vi "VI.OpenRef.caller.vi"(6 "options":i32, 8 "error in":errorcluster caption="error in (no error)", 9 "VI.ref":refnum<vi> caption="VI.ref ('caller' if not wired)") -> (0 "error out":errorcluster, 1 "VI.ref out":refnum<vi>, 4 "opened new?":bool)   [LabVIEW 2020]
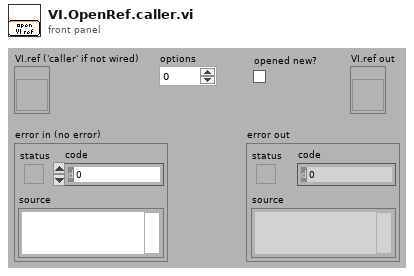
[diagram p1: front panel]
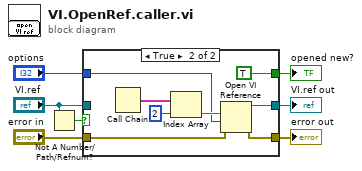
[diagram p0: block diagram]
diagram:
  n1 = Not A Number/Path/Refnum?(number/path/refnum="VI.ref") -> (NaN/Path/Refnum?=w7:bool)
  n2 = case shown="True" w7 {
    tunnel: "VI.ref" -> [w9 _]
    tunnel: [w9 w14] -> w5
    tunnel: [w8 w13] -> w4
    tunnel: "error in" -> [w8 w12]
    tunnel: "options" -> [_ w11]
    tunnel: [_ TRUE] -> w1
    frame False {
    }
    frame True {
      n3 = Call Chain() -> (call chain=w17:string[])
      n4 = Index Array(array=w17, index=2) -> (element=w16:string)
      n5 = Open VI Reference(vi path=w16, options=w11, error in (no error)=w12) -> (vi reference=w14:refnum<vi>, error out=w13:errorcluster)  [unwired: 3 out]
    }
  }
  "VI.ref out" <- w5
  "error out" <- w4
  "opened new?" <- w1
